vi "Periodic String Filter.vi"(0 "Input String":string, 1 "Reset?":bool, 2 "State":T2, 5 "Parameter":string, 9 "Remove Immediately? (F)":bool, 11 "Settings":T3={"threashold(#/s)"=1.0, "Check Peroid(s)"=1.0}, 12 "Level (Normal)":T1) -> (3 "Current Time":timestamp, 4 "Input String (Dup)":string, 10 "Additional Info":string[](array[string]), 14 "Filtered Status":string[](array[string]), 15 "Filtered?":bool)   [LabVIEW 2017, in "Communicable State Machine.lvlib"]
uses:
  Communicable State Machine.lvlib
  Periodic String Filter Setting.ctl
  Periodic String Filter State.ctl
  _support/Periodic String Filter Level.ctl
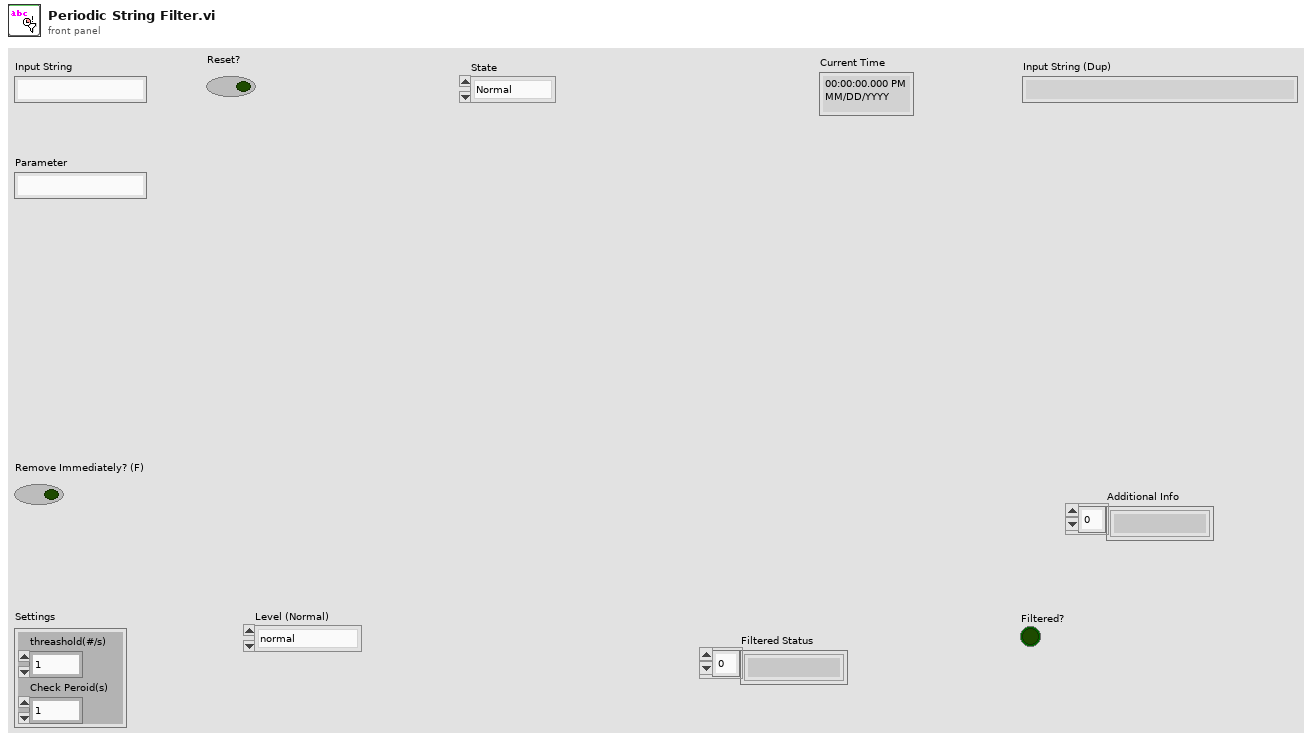
[diagram p1: front panel]
types:
  T1 = typedef "Communicable State Machine.lvlib/Periodic String Filter Level.ctl" = enum16{"normal", "L1", "L2", "L3", "L4"}
  T2 = typedef "Communicable State Machine.lvlib/Periodic String Filter State.ctl" = enum16{"Normal", "Remove All Filters"}
  T3 = typedef "Communicable State Machine.lvlib/Periodic String Filter Setting.ctl" = cluster{"threashold(#/s)":dbl, "Check Peroid(s)":dbl}
  T4 = typedef "Communicable State Machine.lvlib/Periodic String Filter Data.ctl" = cluster{"Keys":string[], "Count":i64[], "LastCheckT":timestamp[], "LastCheckN":i64[], "Filtered":cluster{"Keys":string[], "StartingCount":i64[], "entry":T5[]}}
  T5 = typedef "Communicable State Machine.lvlib/Periodic String Filter Info.ctl" = cluster{"String":string, "Count":i64, "since":timestamp, "param":string, "speed":dbl}
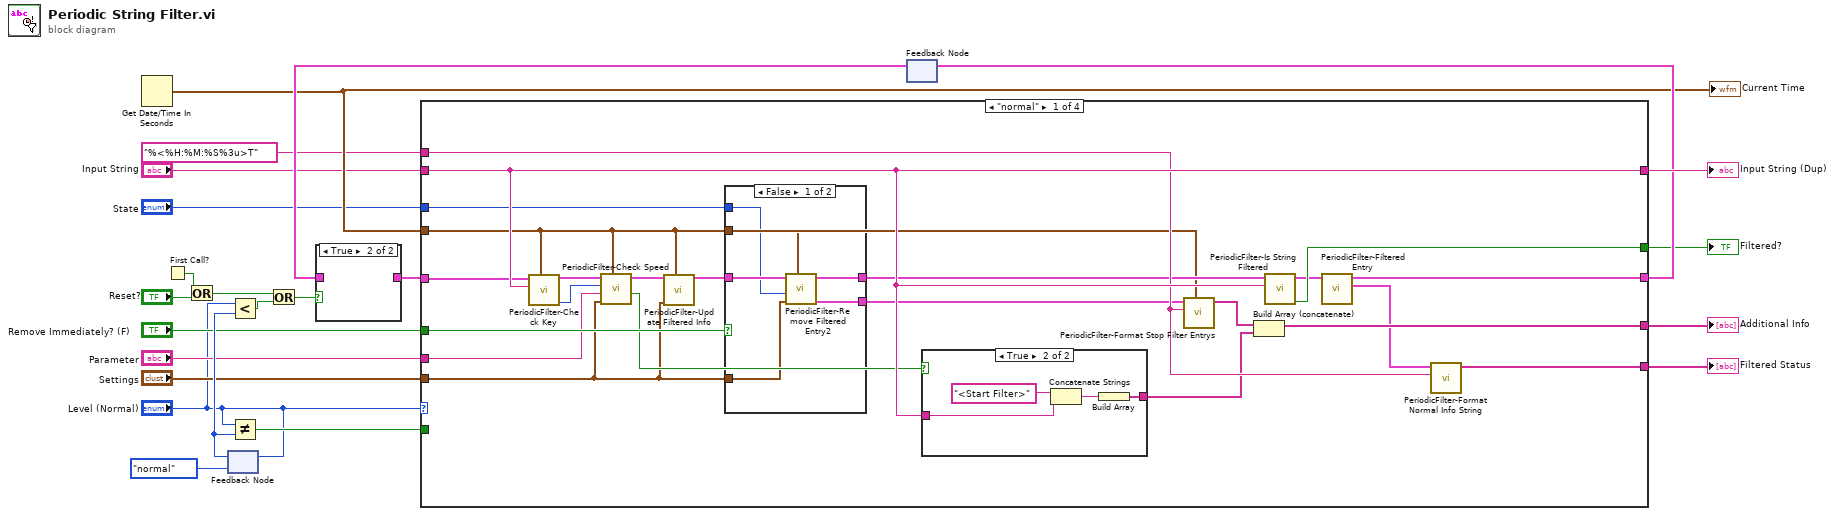
[diagram p0: block diagram]
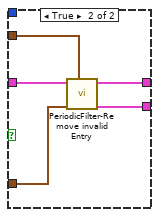
[diagram p2: hidden frame]
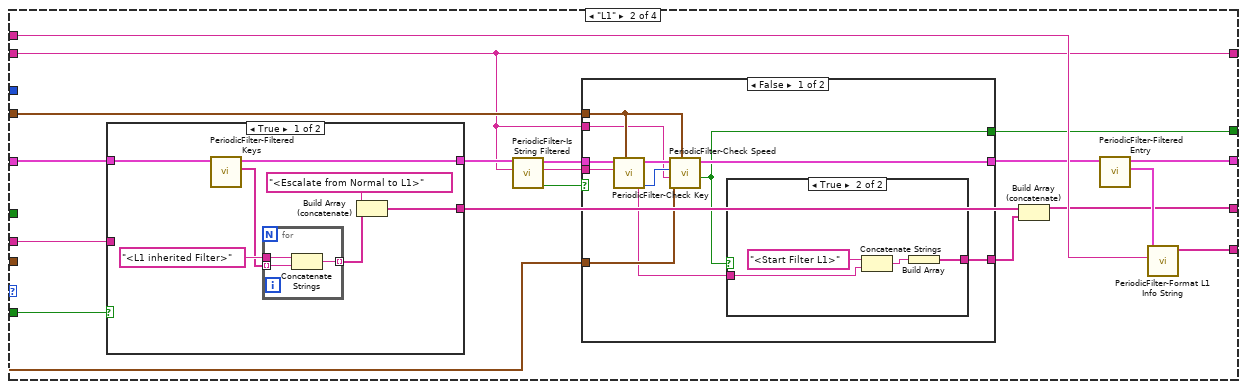
[diagram p4: hidden frame]
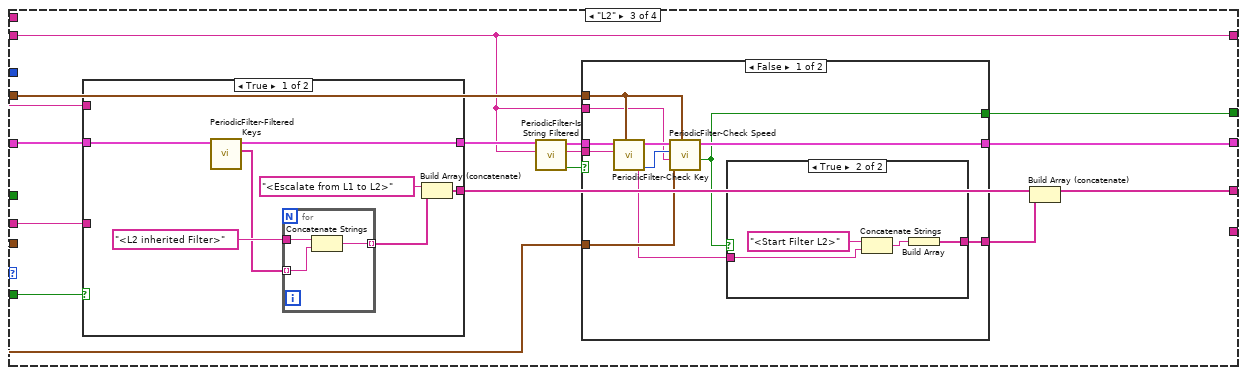
[diagram p8: hidden frame]
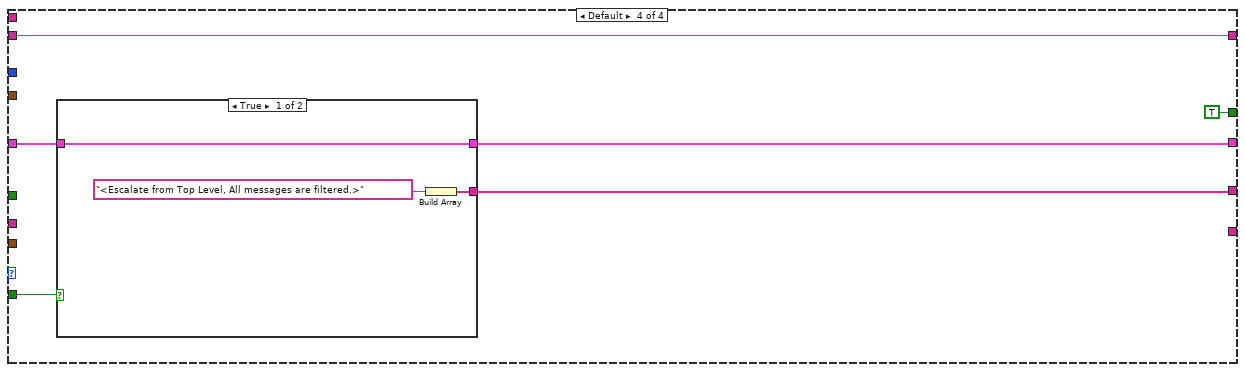
[diagram p12: hidden frame]
diagram:
  n1 = Get Date/Time In Seconds() -> (seconds since 1Jan1904=w12:timestamp)
  "Current Time" <- w12
  n2 = First Call?() -> (First Call?: T/F=w23:bool)
  n3 = Or(x=w23, y="Reset?") -> (x .or. y?=w21:bool)
  n4 = feedback #1(Periodic_String_Filter_Level."normal" ("Level(Normal)")) -> (w18:T1)
  n5 = feedback-in #1("Level (Normal)") -> ()
  n6 = Less?(x="Level (Normal)", y=w18) -> (x < y?=w17:bool)
  n7 = Not Equal?(x="Level (Normal)", y=w18) -> (x != y?=w8:bool)
  n8 = Or(x=w21, y=w17) -> (x .or. y?=w20:bool)
  n9 = feedback #2() -> (w19:T4)  [unwired: 1 in]
  n10 = case shown="True" w20 {
    tunnel: [w24 _] -> w13
    tunnel: w19 -> [w24 _]
    frame False {
    }
    frame True {
    }
  }
  n11 = case shown="\"normal\"" "Level (Normal)" {
    tunnel: "Input String" -> [w47 w63 w109 w156]
    tunnel: [w47 w63 w109 w156] -> w15
    tunnel: "Settings" -> [w26 w67 w113 _]
    tunnel: w12 -> [w25 w68 w114 _]
    tunnel: [w45 w74 w116 w152] -> w14
    tunnel: w13 -> [w44 w81 w123 w154]
    tunnel: [w43 w66 w112 TRUE ("new filtered Item")] -> w9
    tunnel: "Remove Immediately? (F)" -> [w46 _ _ _]
    tunnel: w8 -> [_ w80 w122 w153]
    tunnel: "Parameter" -> [w42 w79 w121 _]
    tunnel: "State" -> [w41 _ _ _]
    tunnel: [w40 w78 _ _] -> w2
    tunnel: [w39 w65 w111 w151] -> w3
    tunnel: "%<%H:%M:%S%3u>T" ("Time format string") -> [w38 w77 _ _]
    frame "normal" {
      n12 = call "PeriodicFilter-Check Key.vi"("Seconds Since 1Jan1904 2"=w25, "Key"=w47, "Data In"=w44) -> ("Index"=w37:i32, "Data Out"=w36:T4)  [unwired: 7 in]
      n13 = call "PeriodicFilter-Check Speed.vi"("Seconds Since 1Jan1904"=w25, "Settings"=w26, "Parameter"=w42, "Index"=w37, "Data In"=w36) -> ("New Filtered Item"=w33:bool, "Data Out"=w35:T4)  [unwired: 4 in, 1 out]
      n14 = call "PeriodicFilter-Update Filtered Info.vi"("Seconds Since 1Jan1904"=w25, "Settings"=w26, "Data In"=w35) -> ("Data Out"=w34:T4)  [unwired: 8 in]
      n15 = case shown="False" w46 {
        tunnel: w34 -> [w53 w58]
        tunnel: w25 -> [w52 w57]
        tunnel: [w51 w56] -> w32
        tunnel: [w50 w55] -> w31
        tunnel: w26 -> [w48 w54]
        tunnel: w41 -> [w49 _]
        frame False {
          n16 = call "PeriodicFilter-Remove Filtered Entry2.vi"("Seconds Since 1Jan1904 2"=w52, "Settings"=w48, "State"=w49, "Data In"=w53) -> ("Removed Info"=w50:T5[], "Data Out"=w51:T4)  [unwired: 6 in]
        }
        frame True {
          n17 = call "PeriodicFilter-Remove invalid Entry.vi"("Seconds Since 1Jan1904 2"=w57, "Settings"=w54, "Data In"=w58) -> ("Removed Info"=w55:T5[], "Data Out"=w56:T4)  [unwired: 7 in]
        }
      }
      n18 = case shown="True" w33 {
        tunnel: [_ w62] -> w28
        tunnel: w47 -> [_ w60]
        frame False {
        }
        frame True {
          n19 = Concatenate Strings("<Start Filter>" ("Current State"), w60) -> (w59:string)
          n20 = Build Array(w59) -> (w62:string[])
        }
      }
      n21 = call "PeriodicFilter-Format Stop Filter Entrys.vi"("Seconds Since 1Jan1904 2"=w25, "Time Format String"=w38, "Removed Info"=w31) -> ("Array"=w27:string[])  [unwired: 8 in]
      n22 = Build Array (concatenate)(w27, w28) -> (w39:string[])
      n23 = call "PeriodicFilter-Is String Filtered.vi"("Input String"=w47, "Data In"=w32) -> ("Filtered"=w43:bool, "Data Out"=w30:T4)  [unwired: 7 in, 1 out]
      n24 = call "PeriodicFilter-Filtered Entry.vi"("Data In"=w30) -> ("Entry"=w29:T5[], "Data Out"=w45:T4)  [unwired: 9 in]
      n25 = call "PeriodicFilter-Format Normal Info String.vi"("Time Format String"=w38, "Removed Info"=w29) -> ("Array"=w40:string[])  [unwired: 9 in]
    }
    frame "L1" {
      n26 = case shown="True" w80 {
        tunnel: w81 -> [w104 w108]
        tunnel: [w98 w108] -> w69
        tunnel: [w99 _] -> w76
        tunnel: w79 -> [_ _]
        frame True {
          n27 = call "PeriodicFilter-Filtered Keys.vi"("Data In"=w104) -> ("Filtered Keys"=w102:string[], "Data Out"=w98:T4)  [unwired: 9 in]
          n28 = for {
            tunnel: w102 -> [w107] mode=indexing
            tunnel: [w106] -> w100 mode=indexing
            tunnel: "<L1 inherited Filter>" ("Current State") -> [w105]
            n29 = Concatenate Strings(w105, w107) -> (w106:string)
          }
          n30 = Build Array (concatenate)("<Escalate from Normal to L1>" ("Current State"), w100) -> (w99:string[])
        }
        frame False {
        }
      }
      n31 = call "PeriodicFilter-Is String Filtered.vi"("Input String"=w63, "Data In"=w69) -> ("Filtered"=w71:bool, "Input String (Dup)"=w73:string, "Data Out"=w72:T4)  [unwired: 7 in]
      n32 = case shown="False" w71 {
        selector: w71 -> [_ w96]
        tunnel: w72 -> [w89 w97]
        tunnel: [w88 w97] -> w70
        tunnel: w68 -> [w87 _]
        tunnel: w73 -> [w82 _]
        tunnel: [w86 _] -> w64
        tunnel: [w85 w96] -> w66
        tunnel: w67 -> [w84 _]
        tunnel: w63 -> [w83 _]
        frame False {
          n33 = call "PeriodicFilter-Check Key.vi"("Seconds Since 1Jan1904 2"=w87, "Key"=w82, "Data In"=w89) -> ("Index"=w90:i32, "Data Out"=w91:T4)  [unwired: 7 in]
          n34 = call "PeriodicFilter-Check Speed.vi"("Seconds Since 1Jan1904"=w87, "Settings"=w84, "Parameter"=w83, "Index"=w90, "Data In"=w91) -> ("New Filtered Item"=w85:bool, "Data Out"=w88:T4)  [unwired: 4 in, 1 out]
          n35 = case shown="True" w85 {
            tunnel: [_ w92] -> w86
            tunnel: w82 -> [_ w95]
            frame False {
            }
            frame True {
              n36 = Concatenate Strings("<Start Filter L1>" ("Current State"), w95) -> (w93:string)
              n37 = Build Array(w93) -> (w92:string[])
            }
          }
        }
        frame True {
        }
      }
      n38 = Build Array (concatenate)(w76, w64) -> (w65:string[])
      n39 = call "PeriodicFilter-Filtered Entry.vi"("Data In"=w70) -> ("Entry"=w75:T5[], "Data Out"=w74:T4)  [unwired: 9 in]
      n40 = call "PeriodicFilter-Format L1 Info String.vi"("Time Format String"=w77, "Entry"=w75) -> ("Array"=w78:string[])  [unwired: 9 in]
    }
    frame "L2" {
      n41 = case shown="True" w122 {
        tunnel: w123 -> [w146 w150]
        tunnel: [w140 w150] -> w115
        tunnel: w109 -> [_ _]
        tunnel: [w141 _] -> w120
        tunnel: w121 -> [_ _]
        frame True {
          n42 = call "PeriodicFilter-Filtered Keys.vi"("Data In"=w146) -> ("Filtered Keys"=w144:string[], "Data Out"=w140:T4)  [unwired: 9 in]
          n43 = for {
            tunnel: w144 -> [w149] mode=indexing
            tunnel: [w148] -> w142 mode=indexing
            tunnel: "<L2 inherited Filter>" ("Current State") -> [w147]
            n44 = Concatenate Strings(w147, w149) -> (w148:string)
          }
          n45 = Build Array (concatenate)("<Escalate from L1 to L2>" ("Current State"), w142) -> (w141:string[])
        }
        frame False {
        }
      }
      n46 = call "PeriodicFilter-Is String Filtered.vi"("Input String"=w109, "Data In"=w115) -> ("Filtered"=w117:bool, "Input String (Dup)"=w119:string, "Data Out"=w118:T4)  [unwired: 7 in]
      n47 = case shown="False" w117 {
        selector: w117 -> [_ w138]
        tunnel: w118 -> [w131 w139]
        tunnel: [w130 w139] -> w116
        tunnel: w114 -> [w129 _]
        tunnel: w119 -> [w124 _]
        tunnel: [w128 _] -> w110
        tunnel: [w127 w138] -> w112
        tunnel: w113 -> [w126 _]
        tunnel: w109 -> [w125 _]
        frame False {
          n48 = call "PeriodicFilter-Check Key.vi"("Seconds Since 1Jan1904 2"=w129, "Key"=w124, "Data In"=w131) -> ("Index"=w132:i32, "Data Out"=w133:T4)  [unwired: 7 in]
          n49 = call "PeriodicFilter-Check Speed.vi"("Seconds Since 1Jan1904"=w129, "Settings"=w126, "Parameter"=w125, "Index"=w132, "Data In"=w133) -> ("New Filtered Item"=w127:bool, "Data Out"=w130:T4)  [unwired: 4 in, 1 out]
          n50 = case shown="True" w127 {
            tunnel: [_ w134] -> w128
            tunnel: w124 -> [_ w137]
            frame False {
            }
            frame True {
              n51 = Concatenate Strings("<Start Filter L2>" ("Current State"), w137) -> (w135:string)
              n52 = Build Array(w135) -> (w134:string[])
            }
          }
        }
        frame True {
        }
      }
      n53 = Build Array (concatenate)(w120, w110) -> (w111:string[])
    }
    frame Default {
      n54 = case shown="True" w153 {
        tunnel: w154 -> [w157 w160]
        tunnel: [w157 w160] -> w152
        tunnel: [w158 _] -> w151
        frame True {
          n55 = Build Array("<Escalate from Top Level, All messages are filtered.>" ("Current State")) -> (w158:string[])
        }
        frame False {
        }
      }
    }
  }
  "Filtered?" <- w9
  "Input String (Dup)" <- w15
  "Additional Info" <- w3
  "Filtered Status" <- w2
  n56 = feedback-in #2(w14) -> ()
